vi "RT.vi"() -> ()   [LabVIEW 2020]
uses:
  <vilib>/FPGAPlugInAG/cRIO-9054/niLvFpga_Open_cRIO-9054.vi
  <vilib>/Utility/error.llb/Error Cluster From Error Code.vi
  <vilib>/FPGAPlugInAG/cRIO-9054/niLvFpga_Reset_cRIO-9054.vi
  <vilib>/FPGAPlugInAG/cRIO-9054/niLvFpga_Run_cRIO-9054.vi
  <vilib>/rvi/errors/niLvFpgaAdjustHostInterfaceError.vi
  <vilib>/FPGAPlugInAG/cRIO-9054/niLvFpga_Close_cRIO-9054.vi
  <vilib>/rvi/interface/nirviOpenFPGA/nirviOpenFPGA.xnode
  FPGA Bitfiles/basiclogging-fpg_FPGATarget2_FPGA_HhNY0sb9fhA.lvbitx
  FPGA.vi
  <vilib>/rvi/interface/nirviMethod/nirviMethod.xnode
  <vilib>/rvi/interface/nirviReadWriteControl/nirviReadWriteControl.xnode
  <vilib>/rvi/interface/nirviCloseFPGA/nirviCloseFPGA.xnode
  <vilib>/rvi/errors/niLvFpgaMergeErrorWithErrorCode.vi
  <vilib>/FPGAPlugInAG/cRIO-9054/niLvFpga_ReadFifo_cRIO-9054.vi
  NiFpgaLv.dll
  <vilib>/FPGAPlugInAG/cRIO-9054/niLvFpga_StartFifo_cRIO-9054.vi
panel:
  out "Data":fxp<+/-,24,7>[](array[numeric])
  out "Waveform Chart":dbl[](graph)
  in  "Loop rate (uSec)":u32=500
  out "Elements Remaining":u32
  out "error out":errorcluster
  out "Timed Out?":bool
  in  "stop":bool
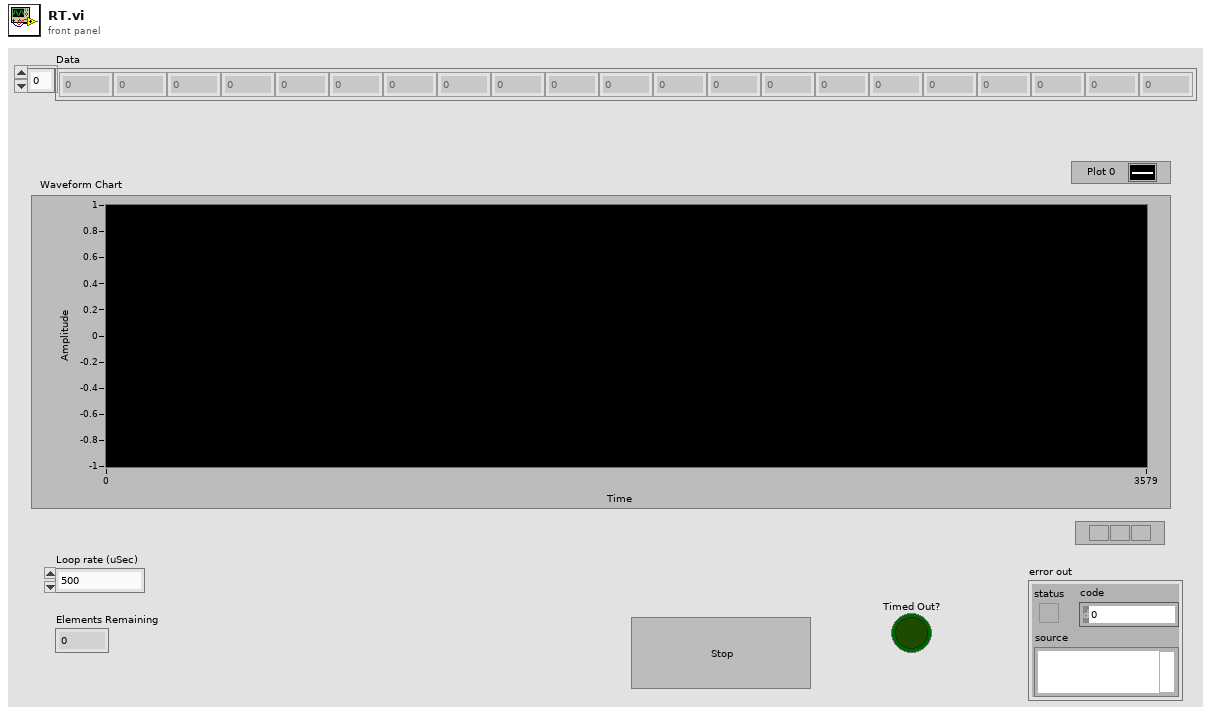
[diagram p1: front panel]
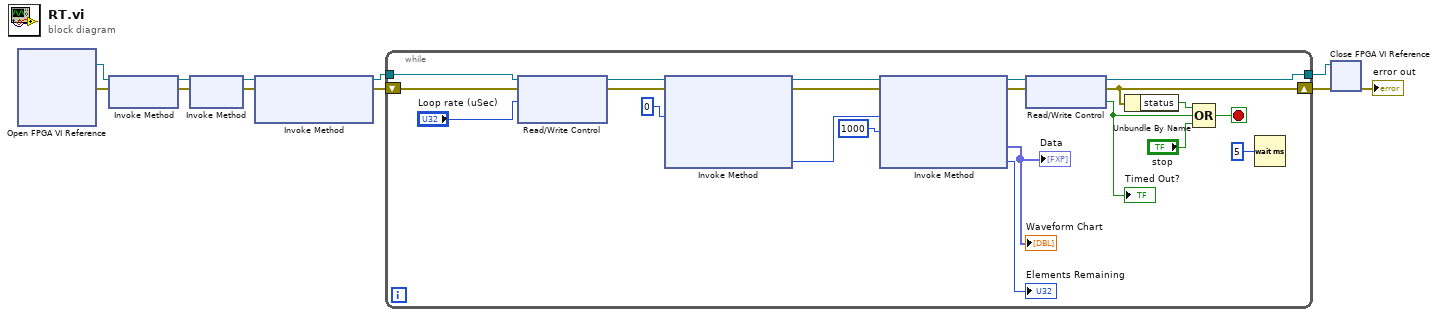
[diagram p0: block diagram]
diagram:
  n1 = xnode "Open FPGA VI Reference"() -> ("FPGA VI Reference Out"=w9:refnum<k20>, "error out"=w8:errorcluster)  [unwired: 2 in]
  n2 = xnode "Invoke Method"("FPGA VI Reference In"=w9, "error in"=w8) -> ("FPGA VI Reference Out"=w4:refnum<k20>, "error out"=w3:errorcluster)
  n3 = xnode "Invoke Method"("FPGA VI Reference In"=w4, "error in"=w3) -> ("FPGA VI Reference Out"=w2:refnum<k20>, "error out"=w1:errorcluster)
  n4 = xnode "Invoke Method"("FPGA VI Reference In"=w2, "error in"=w1) -> ("FPGA VI Reference Out"=w11:refnum<k20>, "error out"=w10:errorcluster)  [unwired: 1 in]
  n5 = while {
    tunnel: w11 -> [w21]
    tunnel: [w31] -> w7
    shift-right: [w25] -> w5
    shift-left: w10 -> [w20]
    stop <- w30 stop-if-true
    n6 = xnode "Read/Write Control"("FPGA VI Reference In"=w21, "error in"=w20, "Rate (uSec) 2"="Loop rate (uSec)") -> ("FPGA VI Reference Out"=w18:refnum<k20>, "error out"=w17:errorcluster)  [unwired: 1 out]
    n7 = xnode "Invoke Method"("FPGA VI Reference In"=w18, "error in"=w17, "Number of Elements"=u32 0) -> ("FPGA VI Reference Out"=w16:refnum<k20>, "error out"=w15:errorcluster, "Elements Remaining"=w14:u32)  [unwired: 1 in, 1 out]
    n8 = xnode "Invoke Method"("FPGA VI Reference In"=w16, "error in"=w15, "Number of Elements"=w14, "Timeout (ms)"=1000) -> ("FPGA VI Reference Out"=w28:refnum<k20>, "error out"=w23:errorcluster, "Data"=→"Waveform Chart" →"Data":fxp<+/-,24,7>[], "Elements Remaining"=→"Elements Remaining":u32)
    n9 = xnode "Read/Write Control"("FPGA VI Reference In"=w28, "error in"=w23) -> ("FPGA VI Reference Out"=w31:refnum<k20>, "error out"=w25:errorcluster, "Timed Out?"=w24:bool)
    "Timed Out?" <- w24
    n10 = Unbundle By Name(w25) -> ("status"=w27:bool)
    n11 = Compound Arithmetic op=OR(w27, w24, "stop") -> (w30:bool)
    n12 = Wait (ms)(milliseconds to wait=u32 5) -> ()  [unwired: 1 out]
  }
  n13 = xnode "Close FPGA VI Reference"("FPGA VI Reference In"=w7, "error in"=w5) -> ("error out"=→"error out":errorcluster)
